vi "FTW-HTTPClient-OpenConnection.vi"(0 "Username":string, 5 "Password":string, 7 "Timeout (10000msec)":i32=10000, 9 "Trusted Server CA Certificate":path, 11 "error in":errorcluster, 12 "Verify Server Certificate?":bool=TRUE) -> (4 "HTTP Client":refnum<class "FTW-HTTPClient.lvclass">, 15 "error out":errorcluster)   [LabVIEW 2015, in "FTW-HTTPClient.lvclass"]
uses:
  FTW-HTTPClient.lvclass
  FTW-HTTPClient.lvclass/FTW-HTTPClient.ctl
  error/FTW-ERR-CallChain.vi
  error/FTW-ERR-NoErrorConstant.vi
  string/FTW-STR-ReplaceWhitespace.vi
  string/FTW-STR-Array-Delimit.vi
  error/FTW-ERR-Clear.vi
  regex/FTW-Regex-ReplaceAll.vi
panel:
  # "Inputs"
  # "Outputs"
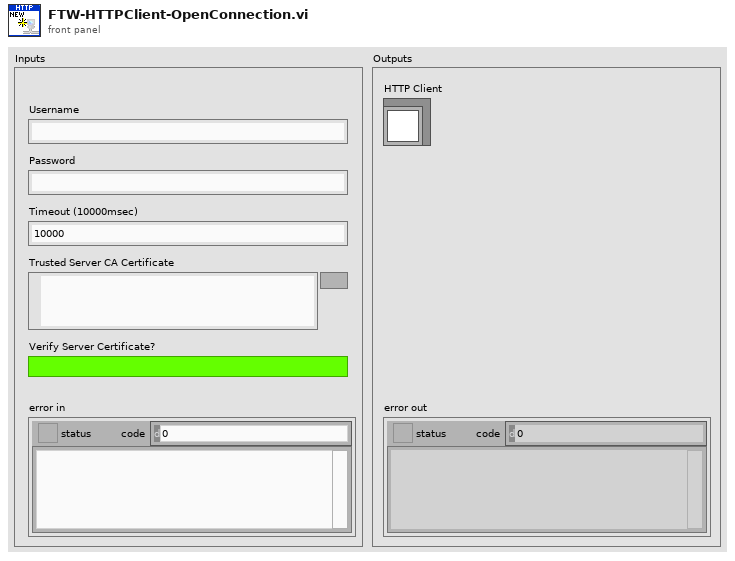
[diagram p1: front panel]
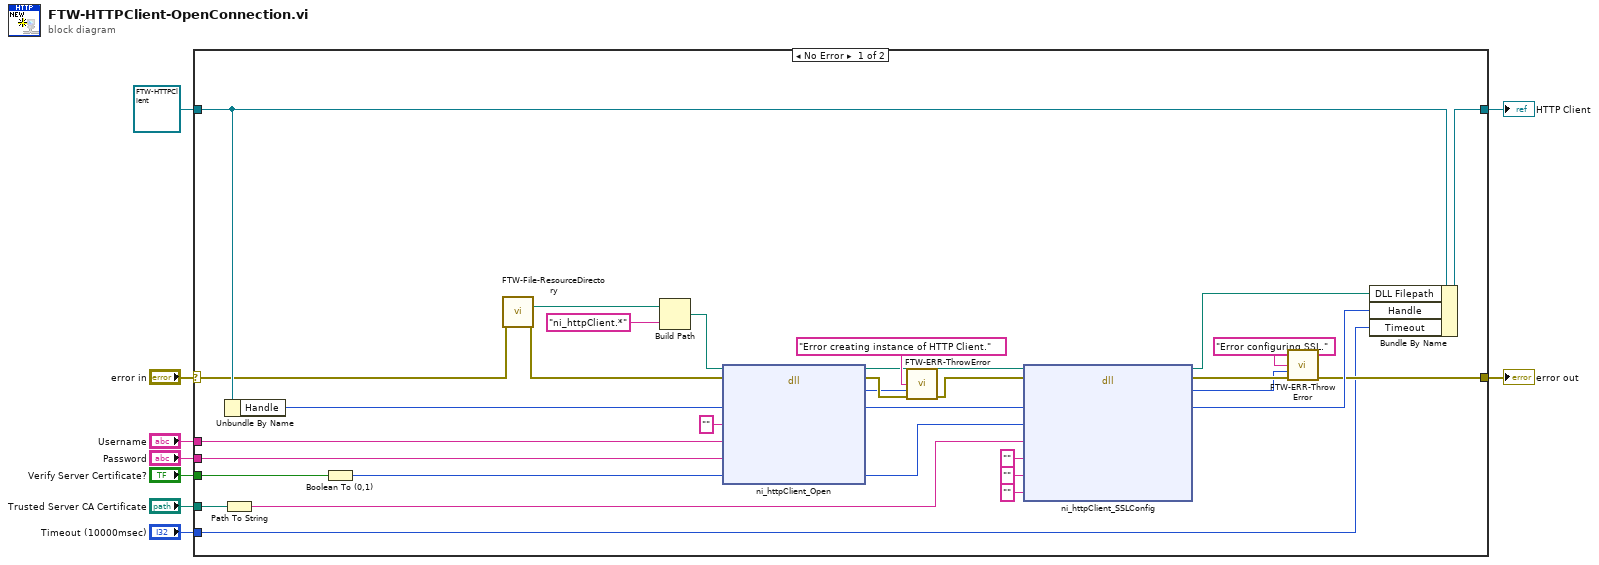
[diagram p0: block diagram]
diagram:
  n1 = case shown="No Error" "error in" {
    selector: "error in" -> [w11 w43]
    tunnel: "Username" -> [w38 _]
    tunnel: "Password" -> [w37 _]
    tunnel: [w25 w43] -> w7
    tunnel: refnum<class "FTW-HTTPClient.lvclass"> refnum ("HTTP Client") -> [w36 w42]
    tunnel: "Trusted Server CA Certificate" -> [w22 _]
    tunnel: [w41 w42] -> w4
    tunnel: "Timeout (10000msec)" -> [w13 _]
    tunnel: "Verify Server Certificate?" -> [w17 _]
    frame No Error {
      n2 = Path To String(path=w22) -> (string=w21:string)
      n3 = Unbundle By Name(w36) -> ("Handle"=w35:u32)
      n4 = Boolean To (0,1)(Boolean=w17) -> (0, 1=w15:i16)
      n5 = call "FTW-File-ResourceDirectory.vi"("error in"=w11) -> ("Resource"=w40:path, "error out"=w10:errorcluster)  [unwired: 10 in, 3 out]
      n6 = Build Path(base path=w40, name or relative path="ni_httpClient.*") -> (appended path=w34:path)
      n7 = dll-call lib="?" fn="ni_httpClient_Open"(path in=w34, error in=w10, "Handle"=w35, "Cookie Filepath"="", "Username"=w38, "Password"=w37, "Verify Server"=w15) -> (path out=w14:path, error out=w33:errorcluster, "Return"=w32:i32, "Handle"=w28:u32, "Verify Server"=w16:i32)  [unwired: 4 in]
      n8 = call "FTW-ERR-ThrowError.vi"("Error Message"="Error creating instance of HTTP Client.", "Error Code"=w32, "error in"=w33) -> ("error out"=w30:errorcluster)  [unwired: 12 in]
      n9 = dll-call lib="?" fn="ni_httpClient_SSLConfig"(path in=w14, error in=w30, "Handle"=w28, "Verify Server"=w16, "CA Cert Filepath"=w21, "Private Key Filepath"="", "Private Key Password"="", "Client Cert Filepath"="") -> (path out=w29:path, error out=w26:errorcluster, "Return"=w24:i32, "Handle"=w27:u32)  [unwired: 6 in]
      n10 = call "FTW-ERR-ThrowError.vi"("Error Message"="Error configuring SSL.", "Error Code"=w24, "error in"=w26) -> ("error out"=w25:errorcluster)  [unwired: 12 in]
      n11 = Bundle By Name(cluster=w36, "DLL Filepath"=w29, "Handle"=w27, "Timeout"=w13) -> (w41:refnum<class "FTW-HTTPClient.lvclass">)
    }
    frame Error {
    }
  }
  "error out" <- w7
  "HTTP Client" <- w4
